vi "Actualizar_DB_parametros.vi"() -> ()   [LabVIEW 2019, in "HMI Class 3.lvclass"]
uses:
  HMI Class 3.lvclass
  HMI Class 3.lvclass/HMI Class 3.ctl
  <vilib>/addons/database/Connection.llb/DB Tools Open Connec (Path).vi
  <vilib>/addons/database/_DB Variant To Data/Database Variant To Data.xnode
  <vilib>/addons/database/NI_Database_API.lvlib
panel:
  out "error out":errorcluster
  in  "error in (no error)":errorcluster
  out "HMI Class 3.lvclass 2":refnum<class "HMI Class 3.lvclass">
  in  "HMI Class 3.lvclass":refnum<class "HMI Class 3.lvclass">
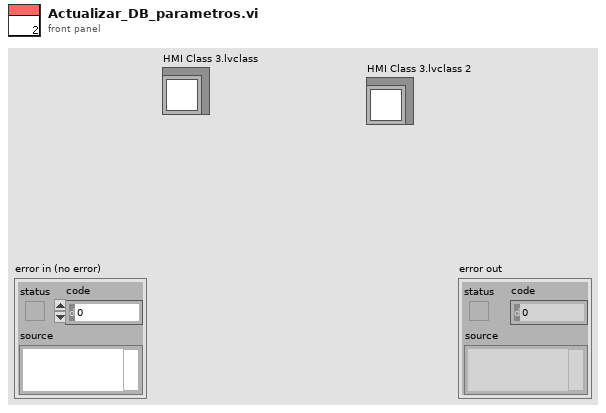
[diagram p1: front panel]
types:
  T1 = typedef "NI_Database_API.lvlib/Conn ObjectReference.ctl" = refnum<k1>
  T2 = cluster{"MODELO":string, "TENSION_MAX":i8, "TENSION_MAX":i8, "TENSION_MAX":i8, "TENSION_MAX":i8, "TENSION_MAX":i8, "TENSION_MAX":i8}
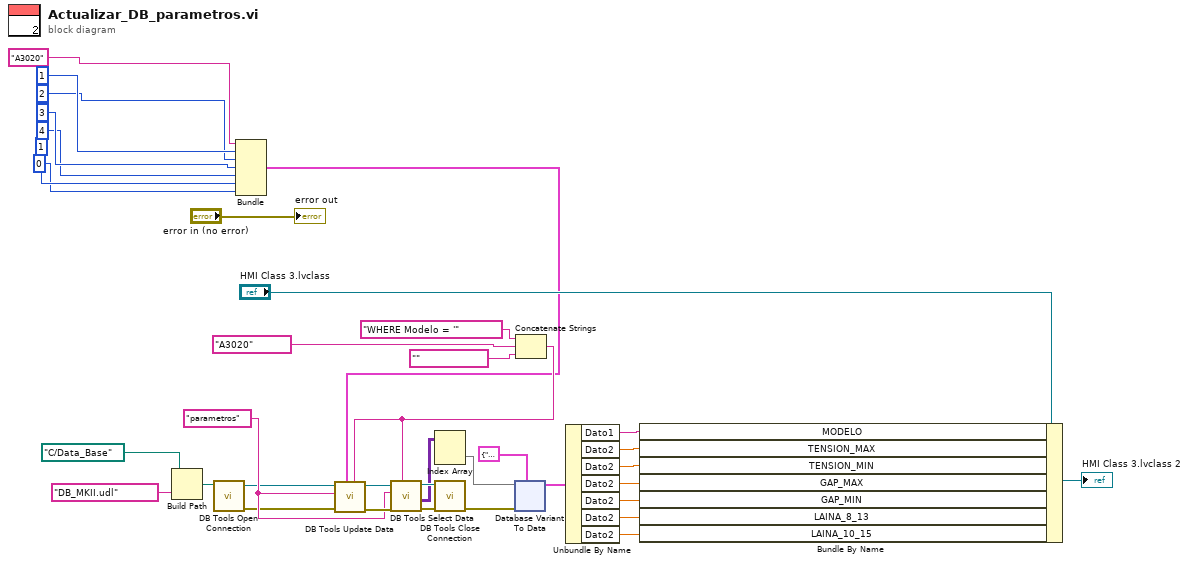
[diagram p0: block diagram]
diagram:
  w12 = "parametros" ("table")
  n1 = Build Path(base path=path "C:/Data_Base", name or relative path="DB_MKII.udl") -> (appended path=w30:path)
  n2 = call-poly <vilib>:"DB Tools Open Connection.vi"("connection information"=w30) -> ("error out"=w11:errorcluster, "connection reference"=w10:T1)  [unwired: 7 in]
  n3 = Bundle("MODELO"="A3020", "TENSION_MAX"=i8 1, "TENSION_MAX"=i8 2, "TENSION_MAX"=i8 3, "TENSION_MAX"=i8 4, "TENSION_MAX"=i8 1, "TENSION_MAX"=i8 0) -> (w9:T2)  [unwired: 1 in]
  n4 = Concatenate Strings("WHERE Modelo = '" ("string"), "A3020" ("string"), "" ("string")) -> (w13:string)
  n5 = call <vilib>:"DB Tools Update Data.vi"("condition"=w13, "data"=w9, "error in (no error)"=w11, "table"=w12, "connection reference"=w10) -> ("error out"=w14:errorcluster, "connection reference out"=w15:T1)  [unwired: 5 in]
  n6 = call <vilib>:"DB Tools Select Data.vi"("condition"=w13, "error in (no error)"=w14, "table"=w12, "connection reference"=w15) -> ("error out"=w35:errorcluster, "data"=w33:variant[][], "connection reference out"=w34:T1)  [unwired: 2 in]
  n7 = Index Array(array=w33) -> (element=w32:variant[])  [unwired: 2 in]
  n8 = call <vilib>:"DB Tools Close Connection.vi"("error in (no error)"=w35, "connection reference"=w34) -> ("error out"=w29:errorcluster)  [unwired: 5 in]
  n9 = xnode "Database Variant To Data"("database variant"=w32, "error in (no error)"=w29, "type"=cluster{"Dato1":string, "Dato2":dbl} {"Dato1"="", "Dato2"=0.0} ("Parametros")) -> ("data"=w27:cluster{"Dato1":string, "Dato2":dbl})  [unwired: 1 out]
  n10 = Unbundle By Name(w27) -> ("Dato1"=w25:string, "Dato2"=w24:dbl, "Dato2"=w23:dbl, "Dato2"=w22:dbl, "Dato2"=w21:dbl, "Dato2"=w20:dbl, "Dato2"=w19:dbl)
  n11 = Bundle By Name(cluster="HMI Class 3.lvclass", "MODELO"=w25, "TENSION_MAX"=w24, "TENSION_MIN"=w23, "GAP_MAX"=w22, "GAP_MIN"=w21, "LAINA_8_13"=w20, "LAINA_10_15"=w19) -> (→"HMI Class 3.lvclass 2":refnum<class "HMI Class 3.lvclass">)
  "error out" <- "error in (no error)"
